vi "Temperature Limit.vi"() -> ()   [LabVIEW 2015]
doc: "This VI simulates the acquisition of temperature, graphs the temperature, and notifies the user if the temperature is over the limit."
panel:
  in  "Start":bool
  in  "Delta t (ms)":i32(slide)=400 scale=50.0..500.0
  in  "Stop":bool
  in  "High Limit":dbl=28.0 format="%.2f"
  out "Temperature":cluster{"Temperature":dbl, "High Limit":dbl}(graph)={"Temperature"=85.88749999999999, "High Limit"=80.0}
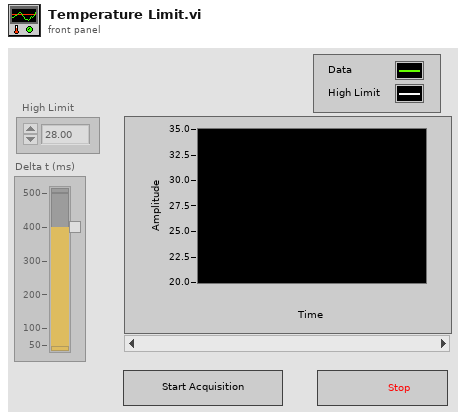
[diagram p1: front panel]
types:
  T1 = cluster{"Temperature Value":dbl, "High Limit":dbl}
  T2 = enum8{"Enabled", "Disabled", "Disabled and Grayed Out"}
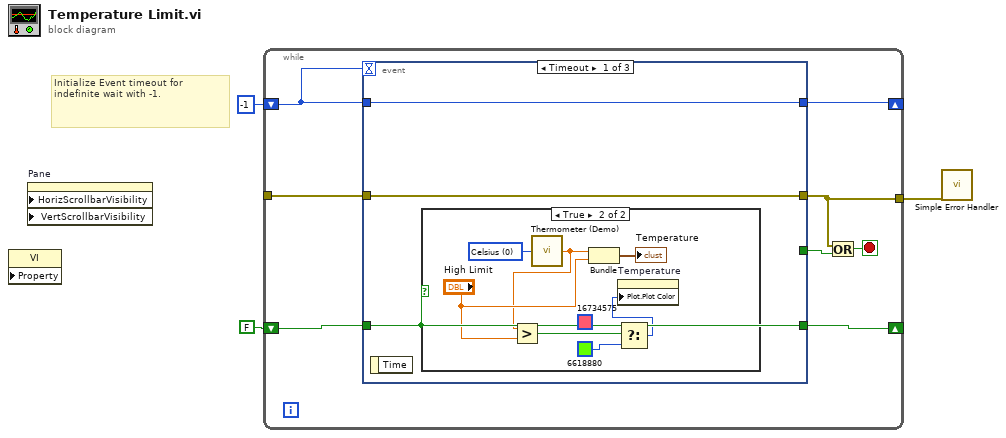
[diagram p0: block diagram]
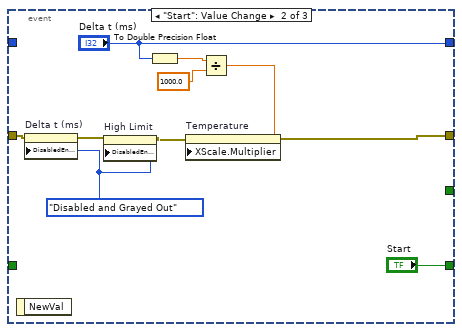
[diagram p3: hidden frame]
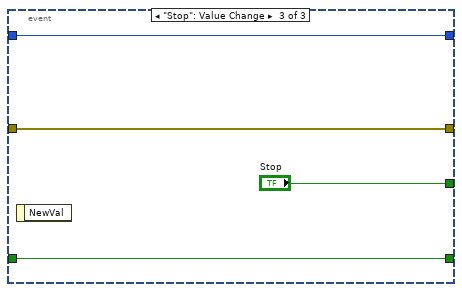
[diagram p4: hidden frame]
diagram:
  # "Initialize Event timeout for indefinite wait with -1."
  n1 = property class="VI" props=[]() -> ()  [unwired: 3 in, 2 out]
  n2 = property on="Pane" class="Pane" props=["HorizScrollbarVisibility", "VertScrollbarVisibility"]() -> ()  [unwired: 4 in, 2 out]
  n3 = while {
    tunnel: [w4] -> _
    tunnel: [w10] -> w2
    shift-right: [w8] -> _
    shift-left: FALSE ("Start") -> [w7]
    shift-right: [w6] -> _
    shift-left: -1 ("Delta t (ms)") -> [w5]
    stop <- w11 stop-if-true
    n4 = event shown="[0] Timeout" {
      selector: _ -> [_ _ _]
      dyn-events: _ -> [_ _ _]
      timeout: w5 -> [_ _ _]
      tunnel: [_ _ "Stop"] -> w9
      tunnel: [w14 w31 w35] -> w4
      tunnel: [w14 w23 w35] -> w10
      tunnel: [w12 "Start" w34] -> w8
      tunnel: w7 -> [w12 _ w34]
      tunnel: [w13 "Delta t (ms)" w33] -> w6
      tunnel: w5 -> [w13 _ w33]
      event Timeout {
        n5 = event-data() -> ()  [unwired: 1 in, 1 out]
        n6 = case shown="True" w12 {
          frame False {
          }
          frame True {
            w21 = u16 0 items=["Celsius", "Fahrenheit"] ("Units (0: Celsius)")
            n7 = call "Thermometer (Demo).vi"("Units (0: Celsius)"=w21) -> ("Temperature Value"=w15:dbl)
            n8 = Greater?(x=w15, y="High Limit") -> (0:w16:bool)
            n9 = Bundle("Temperature Value"=w15, "High Limit"="High Limit") -> (→"Temperature":T1)  [unwired: 1 in]
            n10 = Select(t=u32 16734575, s=w16, f=u32 6618880) -> (s? t:f=w18:u32)
            n11 = property on="Temperature" class="WFChart (strict)"("Plot.Plot Color"=w18) -> ()  [unwired: 2 in, 2 out]
          }
        }
      }
      event "Start": Value Change {
        w24 = T2."Disabled and Grayed Out" ("Disabled")
        n12 = event-data() -> ()  [unwired: 1 in, 1 out]
        n13 = property on="Delta t (ms)" class="Slide (strict)"(error in=w31, "DisabledEnum"=w24) -> (error out=w30:errorcluster)  [unwired: 1 in, 1 out]
        n14 = property on="High Limit" class="DigNum (strict)"(error in=w30, "DisabledEnum"=w24) -> (error out=w29:errorcluster)  [unwired: 1 in, 1 out]
        n15 = To Double Precision Float(number="Delta t (ms)") -> (double precision float=w27:dbl)
        n16 = Divide(x=w27, y=1000.0) -> (x/y=w25:dbl)
        n17 = property on="Temperature" class="WFChart (strict)"(error in=w29, "XScale.Multiplier"=w25) -> (error out=w23:errorcluster)  [unwired: 1 in, 1 out]
      }
      event "Stop": Value Change {
        n18 = event-data() -> ()  [unwired: 1 in, 1 out]
      }
    }
    n19 = Or(x=w10, y=w9) -> (x .or. y?=w11:bool)
  }
  n20 = call <vilib>:"Simple Error Handler.vi"("error in (no error)"=w2) -> ()  [unwired: 4 in, 5 out]
